vi "Electric ECU_Create.vi"(0 "reference in":refnum<class "Electric ECU.lvclass">, 11 "Error In":errorcluster) -> (4 "reference out":refnum<class "Electric ECU.lvclass">, 15 "Error Out":errorcluster)   [LabVIEW 2024, in "Electric ECU.lvclass"]
uses:
  Electric ECU.lvclass/Electric ECU.ctl
  Electric ECU.lvclass
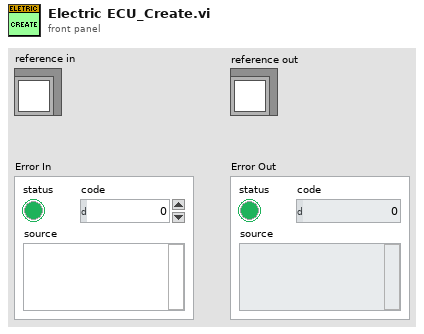
[diagram p1: front panel]
types:
  T1 = typedef "Electric ECU.lvclass/ObjectAttributes.ctl" = cluster{"None":bool}
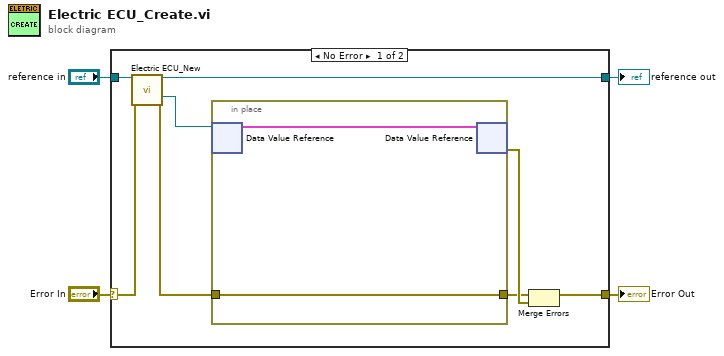
[diagram p0: block diagram]
diagram:
  n1 = case shown="No Error" "Error In" {
    selector: "Error In" -> [w11 w16]
    tunnel: [w5 w16] -> w3
    tunnel: "reference in" -> [w12 w15]
    tunnel: [w10 w15] -> w1
    frame No Error {
      n2 = call "Electric ECU_New.vi"("reference in"=w12, "Error In"=w11) -> ("reference out"=w10:refnum<class "Electric ECU.lvclass">, "DVRRefOut"=w8:refnum<data-value>, "Error Out"=w7:errorcluster)  [unwired: 10 in, 1 out]
      n3 = in-place {
        in-place-border: w7 -> [w13]
        in-place-border: [w13] -> w6
        n4 = in-place-dvr #1(w8) -> (w14:T1)  [unwired: 1 out]
        n5 = in-place-dvr #1(w14) -> (w9:errorcluster)  [unwired: 1 out]
      }
      n6 = Merge Errors(w6, w9) -> (w5:errorcluster)
    }
    frame Error {
      # "VI-TechBaseTemplate_Simple_4x4x4"
    }
  }
  "Error Out" <- w3
  "reference out" <- w1
